vi "Next Segment.vi"(8 "error in (no error)":errorcluster, 10 "Count":i32, 11 "File Response in":refnum<class "File Response.lvclass">) -> (0 "error out":errorcluster, 1 "Last?":bool, 2 "Data":string, 3 "File Response out":refnum<class "File Response.lvclass">)   [LabVIEW 2020, in "HTTP Utils.lvlib" / "File Response.lvclass"]
uses:
  File Response.lvclass
  File Response.lvclass/File Response.ctl
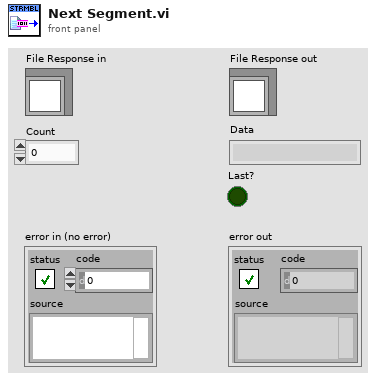
[diagram p1: front panel]
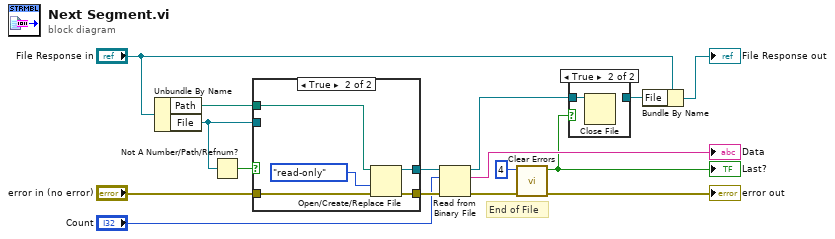
[diagram p0: block diagram]
diagram:
  # "End of File"
  n1 = Unbundle By Name("File Response in") -> ("Path"=w14:path, "File"=w13:refnum<file>)
  n2 = Not A Number/Path/Refnum?(number/path/refnum=w13) -> (NaN/Path/Refnum?=w15:bool)
  n3 = case shown="True" w15 {
    tunnel: w14 -> [_ w23]
    tunnel: w13 -> [w18 _]
    tunnel: [w18 w21] -> w11
    tunnel: "error in (no error)" -> [w17 w20]
    tunnel: [w17 w19] -> w10
    frame False {
    }
    frame True {
      n4 = Open/Create/Replace File(file path (use dialog)=w23, error in=w20, access (0:read/write)=enum16{"read/write", "read-only", "write-only"}."read-only") -> (refnum out=w21:refnum<file>, error out=w19:errorcluster)  [unwired: 3 in, 1 out]
    }
  }
  n5 = Read from Binary File(8:w10, 10:"Count", 11:w11) -> (0:w4:errorcluster, 2:→"Data":string, 3:w6:refnum<file>)  [unwired: 3 in, 1 out]
  n6 = call <vilib>:"Clear Errors.vi"("error in (no error)"=w4, "specific error code to clear (0: all)"=4) -> ("error out"=→"error out":errorcluster, "specific error cleared?"=w1:bool)  [unwired: 4 in]
  "Last?" <- w1
  n7 = case shown="True" w1 {
    tunnel: w6 -> [w24 w25]
    tunnel: [w24 _] -> w5
    frame False {
    }
    frame True {
      n8 = Close File(refnum=w25) -> ()  [unwired: 1 in, 2 out]
    }
  }
  n9 = Bundle By Name(cluster="File Response in", "File"=w5) -> (→"File Response out":refnum<class "File Response.lvclass">)
